vi "VC_UItem.vi"(8 "error in (no error)":errorcluster, 10 "UI Item label":string, 11 "D&C_SchemaBase in":refnum<class "D&C_SchemaBase.lvclass">) -> (0 "error out":errorcluster, 3 "D&C_SchemaBase out":refnum<class "D&C_SchemaBase.lvclass">)   [LabVIEW 2020, in "D&C_SchemaBase.lvlib" / "D&C_SchemaBase.lvclass"]
uses:
  D&C_SchemaBase.lvclass
  D:/Projets/STEP AT/LUGE 2022.2/Demo UIA/support/UI_Actor.lvlibp/UI_Actor/UI_Actor.lvclass
  support/UI_Actor.lvlibp/UI_Actor/UI_Elmt_Ref(Label).vi
  support/UI_Actor.lvlibp/UI_Actor/UI_Actor.lvclass
  D:/Projets/STEP AT/LUGE 2022.2/Demo UIA/support/Actor Framework.lvlibp/1abvi3w/vi.lib/ActorFramework/Actor/Actor.lvclass
  D:/Projets/STEP AT/LUGE 2022.2/Demo UIA/D&Cs/D&C_SchemaBase/D&C_SchemaBase/D&C_SchemaBase.lvclass
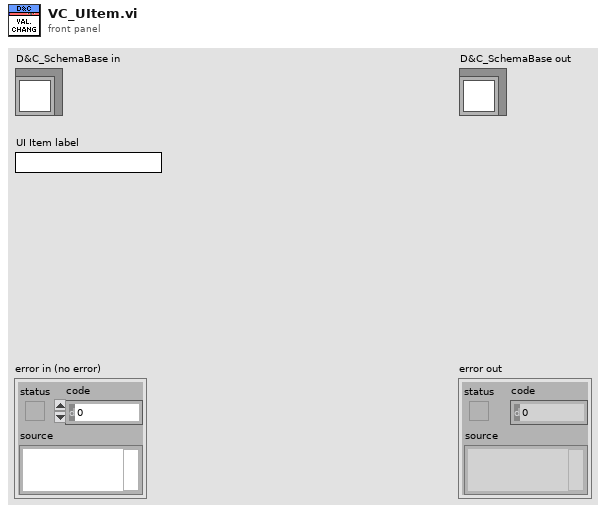
[diagram p1: front panel]
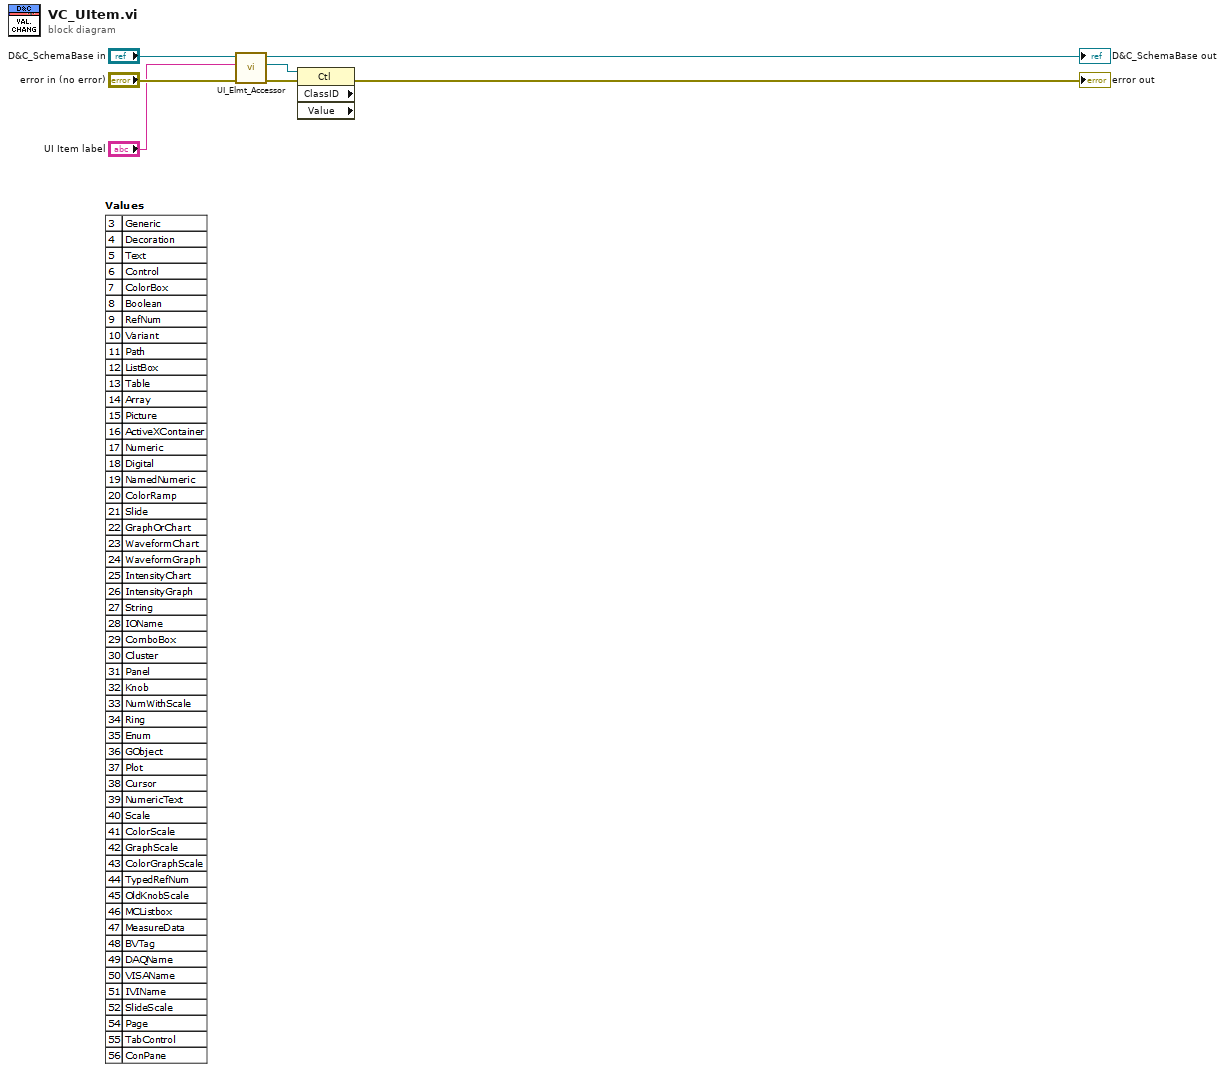
[diagram p0: block diagram]
diagram:
  n1 = call-poly "UI_Elmt_Accessor.vi"("error in (no error)"="error in (no error)", "Elmt Label"="UI Item label", "UI_Actor in"="D&C_SchemaBase in") -> ("error out"=w2:errorcluster, "Ctl Refnum"=w3:refnum<vi>, "UI_Actor out"=→"D&C_SchemaBase out":refnum<class "D&C_SchemaBase.lvclass">)  [unwired: 5 in, 1 out]
  n2 = property class="Ctl" props=["ClassID", "Value"](reference=w3, error in=w2) -> (error out=→"error out":errorcluster)  [unwired: 3 out]
